vi "Setting Average time.vi"(2 "Assign  averexp according to the chart on the right":dbl=4.0, 3 "VISA resource name":refnum<visa-resource-name>="GPIB12::28::INSTR") -> (0 "Read out result":string, 1 "Send string":string)   [LabVIEW 2010]
panel:
  in  "byte count":u32=128
  out "error out":errorcluster {"code" format="%.0x"}
  in  "error in":errorcluster {"code" format="%.0x"}
  # "Average over time: setting the measurement time"
  # "Default setting is 4"
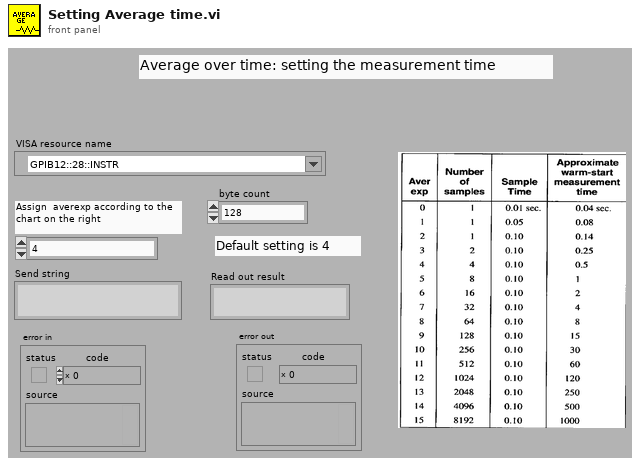
[diagram p1: front panel]
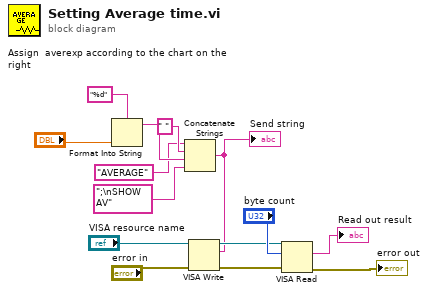
[diagram p0: block diagram]
diagram:
  n1 = Format Into String(format string="%d", "Assign  averexp according to the chart on the right") -> (resulting string=w10:string)  [unwired: 2 in, 1 out]
  n2 = Concatenate Strings("AVERAGE" ("string"), " " ("string"), w10, ";\nSHOW AV" ("format string")) -> (w3:string)
  "Send string" <- w3
  n3 = VISA Write(VISA resource name="VISA resource name", write buffer=w3, error in (no error)="error in") -> (VISA resource name out=w6:refnum<visa-resource-name>, error out=w5:errorcluster)  [unwired: 1 out]
  n4 = VISA Read(VISA resource name=w6, byte count="byte count", error in (no error)=w5) -> (read buffer=→"Read out result":string, error out=→"error out":errorcluster)  [unwired: 2 out]
